vi "Insert new delta region in ramping array_WIP.vi"() -> ()   [LabVIEW 2015]
panel:
  out "Numeric":dbl
  out "Final Array":dbl[](array[numeric])
  out "Insert Index":i32
  out "START":i32
  out "END":i32
  out "HR Array":dbl[](array[numeric])
  in  "Start 2":dbl=0.6
  in  "End 2":dbl=1.1
  in  "Delta 2":dbl=0.1
  in  "OK Button":bool=TRUE
  out "Output Array (1D)":dbl[](array[numeric])
  out "Array length":i32
  out "Error Out":errorcluster
  in  "Start":dbl
  in  "End":dbl=2.0
  in  "Delta":dbl=0.5
  in  "Error In":errorcluster
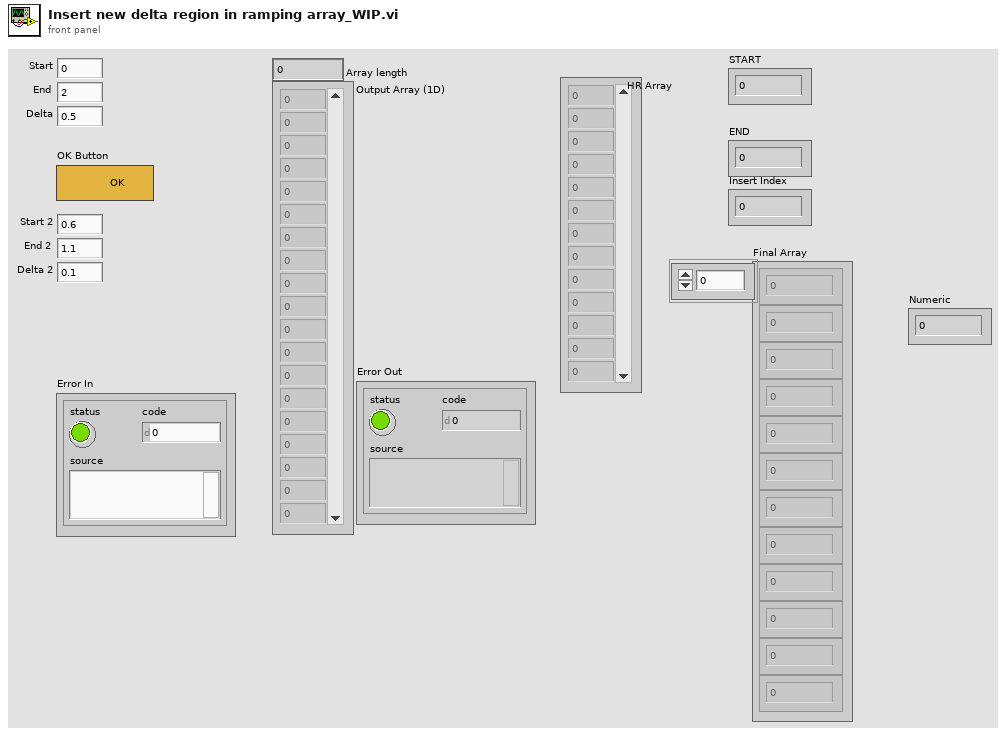
[diagram p1: front panel]
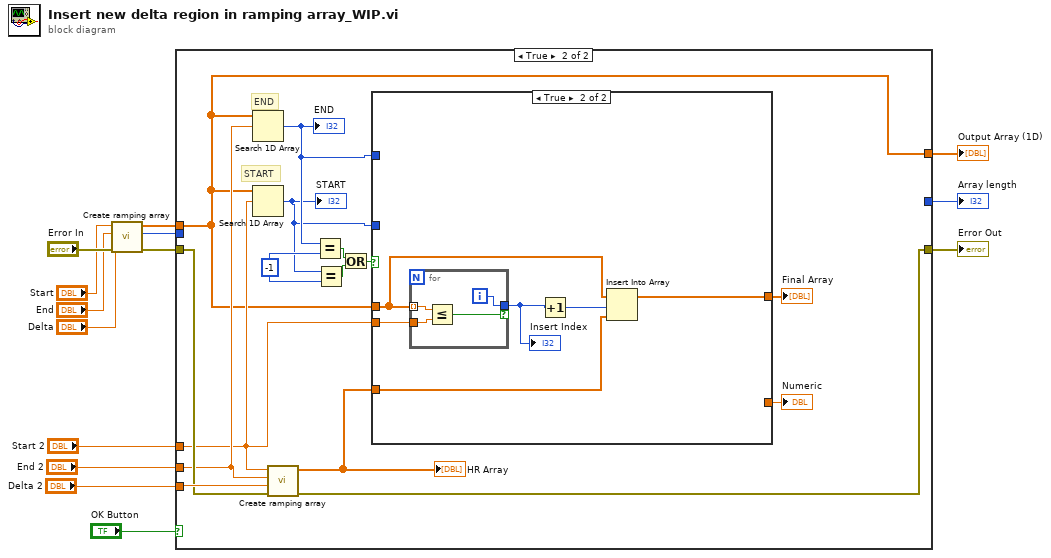
[diagram p0: block diagram]
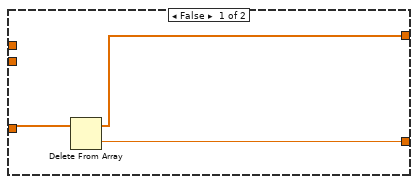
[diagram p3: hidden frame]
diagram:
  n1 = call "Create ramping array.vi"("Error In"="Error In", "Delta"="Delta", "End"="End", "Start"="Start") -> ("Error Out"=w11:errorcluster, "Array length"=w10:i32, "Output Array (1D)"=w9:dbl[])  [unwired: 5 in]
  n2 = case shown="True" "OK Button" {
    tunnel: w11 -> [w17 w31]
    tunnel: w10 -> [w16 _]
    tunnel: w9 -> [w15 w21]
    tunnel: [w17 w30] -> w8
    tunnel: [w16 _] -> w7
    tunnel: [w15 w21] -> w6
    tunnel: "Start 2" -> [_ w24]
    tunnel: "End 2" -> [_ w29]
    tunnel: "Delta 2" -> [_ w32]
    frame False {
    }
    frame True {
      w25 = -1 ("y")
      # "START"
      # "END"
      n3 = Search 1D Array(1D array=w21, element=w29) -> (index of element=w23:i32)  [unwired: 1 in]
      "END" <- w23
      n4 = Search 1D Array(1D array=w21, element=w24) -> (index of element=w22:i32)  [unwired: 1 in]
      "START" <- w22
      n5 = call "Create ramping array.vi"("Error In"=w31, "Delta"=w32, "End"=w29, "Start"=w24) -> ("Error Out"=w30:errorcluster, "Output Array (1D)"=w20:dbl[])  [unwired: 5 in, 1 out]
      "HR Array" <- w20
      n6 = Equal?(x=w23, y=w25) -> (x = y?=w27:bool)
      n7 = Equal?(x=w22, y=w25) -> (x = y?=w26:bool)
      n8 = Or(x=w27, y=w26) -> (x .or. y?=w28:bool)
      n9 = case shown="True" w28 {
        tunnel: w24 -> [_ w41]
        tunnel: w23 -> [_ _]
        tunnel: w22 -> [_ _]
        tunnel: w21 -> [_ w40]
        tunnel: w20 -> [w35 w39]
        tunnel: [w34 w38] -> w19
        tunnel: [w33 _] -> w18
        frame False {
          n10 = Delete From Array(array=w35) -> (deleted portion=w33:dbl, array with subset deleted=w34:dbl[])  [unwired: 2 in]
        }
        frame True {
          n11 = for {
            tunnel: w40 -> [w45] mode=indexing
            tunnel: w41 -> [w44]
            tunnel: [w43] -> w36 if=w42
            i -> [w43]
            n12 = Less Or Equal?(x=w45, y=w44) -> (x <= y?=w42:bool)
          }
          "Insert Index" <- w36
          n13 = Increment(x=w36) -> (x+1=w37:i32)
          n14 = Insert Into Array(array=w40, index=w37, new element=w39) -> (w38:dbl[])
        }
      }
      "Final Array" <- w19
      "Numeric" <- w18
    }
  }
  "Error Out" <- w8
  "Array length" <- w7
  "Output Array (1D)" <- w6
